vi "Close Device.vi"(8 "Error In":errorcluster, 11 "LINX Device Config":T1) -> (0 "Error Out":errorcluster, 3 "LINX Device Config":T1)   [LabVIEW 2011, in "LVH-LINX.lvlib" / "Device.lvlib"]
doc: "Close the connection to the LINX device."
uses:
  <vilib>/LabVIEW Hacker/LINX/Private/Device/Device.lvlib
  Type Defs/LINX Device Config.ctl
  Type Defs/Interface.ctl
  Type Defs/TCP Config.ctl
  Type Defs/Device Family.ctl
  <vilib>/LabVIEW Hacker/LINX/LVH-LINX.lvlib
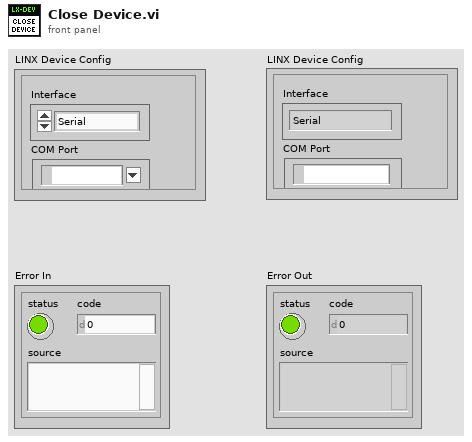
[diagram p1: front panel]
types:
  T1 = typedef "LVH-LINX.lvlib/Device.lvlib/LINX Device Config.ctl" = cluster{"Interface":T2, "COM Port":refnum<visa-resource-name>, "TCP Configuration":T3, "Device ID":u8, "Device Name":string, "Device Family":T4}
  T2 = typedef "LVH-LINX.lvlib/Interface.ctl" = enum16{"Serial", "TCP"}
  T3 = typedef "LVH-LINX.lvlib/Device.lvlib/TCP Config.ctl" = cluster{"IP Address":string, "Port":dbl}
  T4 = typedef "LVH-LINX.lvlib/Device Family.ctl" = enum8{"National Instruments", "Digilent", "Arduino"}
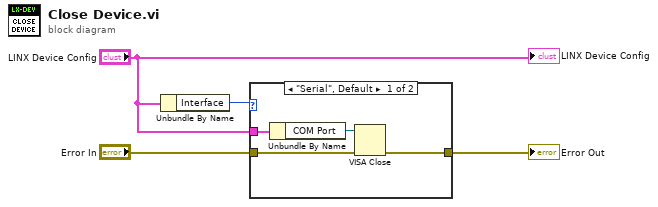
[diagram p0: block diagram]
diagram:
  n1 = Unbundle By Name("LINX Device Config") -> ("Interface"=w2:T2)
  n2 = case shown="\"Serial\", Default" w2 {
    tunnel: "LINX Device Config" -> [w8 _]
    tunnel: "Error In" -> [w6 w9]
    tunnel: [w5 w9] -> w3
    frame "Serial", Default {
      n3 = Unbundle By Name(w8) -> ("COM Port"=w7:refnum<visa-resource-name>)
      n4 = VISA Close(VISA resource name=w7, error in (no error)=w6) -> (error out=w5:errorcluster)
    }
    frame "TCP" {
      # "!!!"
    }
  }
  "Error Out" <- w3
  "LINX Device Config" <- "LINX Device Config"
